vi "Add Sprite.vi"(7 "Point":T1, 8 "Height":i32, 9 "Width":i32, 10 "Sprite Array In":i32[][](array[numeric]), 11 "Pixel Array In":i32[](array[numeric])) -> (3 "Pixel Array Out":i32[](array[numeric]))   [LabVIEW 2019]
doc: "Overlays the white image array elements onto the pixel array, creating a fire 'source'."
uses:
  _2D/Point.ctl
  _2D/2D.lvlib
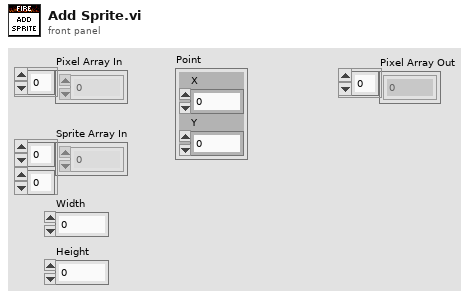
[diagram p1: front panel]
types:
  T1 = typedef "2D.lvlib/Point.ctl" = cluster{"X":i16, "Y":i16}
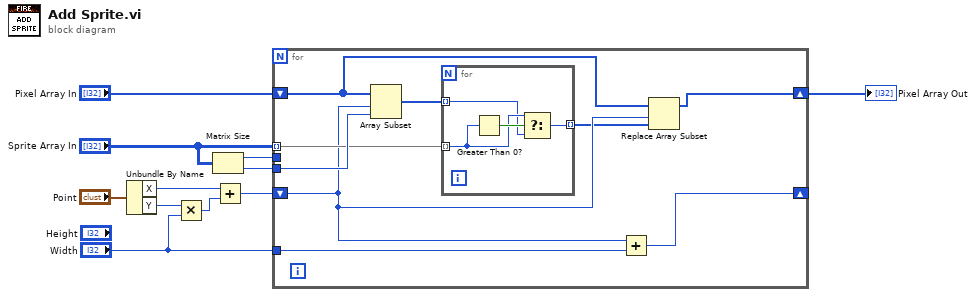
[diagram p0: block diagram]
diagram:
  n1 = Unbundle By Name("Point") -> ("X"=w7:i16, "Y"=w8:i16)
  n2 = Multiply(x=w8, y="Width") -> (x*y=w6:i32)
  n3 = Matrix Size(0:"Sprite Array In") -> (1:w3:i32, 2:w2:i32)
  n4 = Add(x=w7, y=w6) -> (x+y=w5:i32)
  n5 = for {
    tunnel: "Sprite Array In" -> [w16] mode=indexing
    shift-right: [w12] -> w10
    shift-left: "Pixel Array In" -> [w15]
    tunnel: w3 -> [_]
    tunnel: w2 -> [w17]
    shift-right: [w18] -> _
    shift-left: w5 -> [w14]
    tunnel: "Width" -> [w19]
    n6 = Array Subset(array=w15, index=w14, length=w17) -> (w20:i32[])
    n7 = for {
      tunnel: w20 -> [w22] mode=indexing
      tunnel: w16 -> [w23] mode=indexing
      tunnel: [w21] -> w13 mode=indexing
      n8 = Greater Than 0?(x=w23) -> (x > 0?=w24:bool)
      n9 = Select(t=w23, s=w24, f=w22) -> (s? t:f=w21:i32)
    }
    n10 = Add(x=w14, y=w19) -> (x+y=w18:i32)
    n11 = Replace Array Subset(array=w15, new element=w13, index=w14) -> (w12:i32[])
  }
  "Pixel Array Out" <- w10
